vi "Create Command.vi"(10 "Command Queue":refnum<queue>) -> (3 "Play.lvclass":refnum<class "Play.lvclass">)   [LabVIEW 2010, in "Play.lvclass"]
doc: "This instance of Create Command.vi writes the value of the Command Queue reference to the data stored within Play.lvclass."
uses:
  Play.lvclass
  Application Command/Application Command.lvclass
  Play.lvclass/Play.ctl
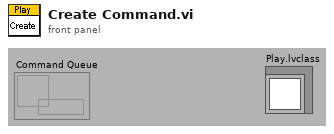
[diagram p1: front panel]
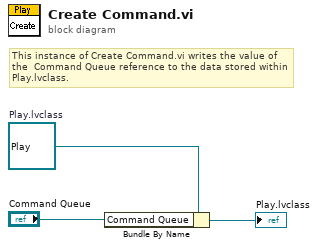
[diagram p0: block diagram]
diagram:
  w3 = refnum<class "Play.lvclass"> refnum  # Play.lvclass
  # "This instance of Create Command.vi writes the value of the  Command Queue reference to the data stored within Play.lvclass."
  n1 = Bundle By Name "Bundle By Name"(cluster=w3, "Command Queue"="Command Queue") -> (→"Play.lvclass":refnum<class "Play.lvclass">)
